vi "Configure Proxy Server.vi"(5 "proxy password":string, 7 "proxy username":string, 8 "error in":errorcluster, 9 "proxy port":u16, 10 "proxy":string, 11 "session in":refnum<class "Session.lvclass">) -> (0 "error out":errorcluster, 3 "session out":refnum<class "Session.lvclass">)   [LabVIEW 2019, in "NI_Advanced HTTP Client.lvlib" / "Session.lvclass"]
doc: "Configures the session to use a proxy server and provides the required login credentials for the proxy."
uses:
  Session.lvclass
  Session.lvclass/Session.ctl
  lvwebclient_32.dll
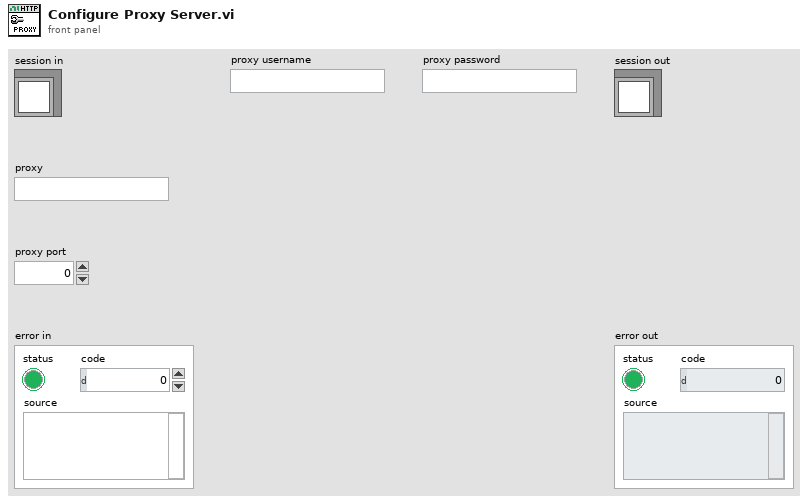
[diagram p1: front panel]
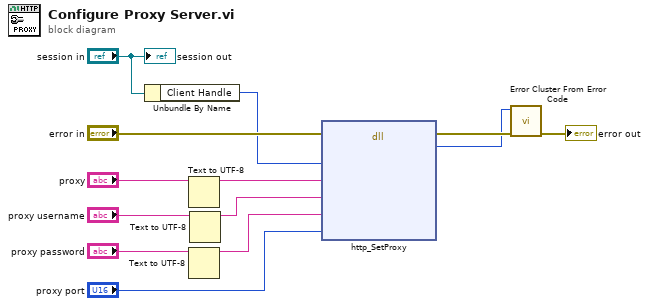
[diagram p0: block diagram]
diagram:
  n1 = Unbundle By Name("session in") -> ("Client Handle"=w8:u32)
  n2 = Text to UTF-8(11:"proxy") -> (3:w6:string)  [unwired: 2 in, 1 out]
  n3 = Text to UTF-8(11:"proxy password") -> (3:w3:string)  [unwired: 2 in, 1 out]
  n4 = Text to UTF-8(11:"proxy username") -> (3:w5:string)  [unwired: 2 in, 1 out]
  n5 = dll-call lib="C:/source/github/ni-adv-http-api/Advanced HTTP Client/lvwebclient_*.*" fn="http_SetProxy"(error in="error in", "handle"=w8, "proxy"=w6, "proxyUser"=w5, "proxyPW"=w3, "proxyPort"="proxy port") -> (error out=w9:errorcluster, "return"=w1:i32)  [unwired: 7 in, 1 out]
  n6 = call <vilib>:"Error Cluster From Error Code.vi"("error in (no error)"=w9, "error code (0)"=w1) -> ("error out"=→"error out":errorcluster)  [unwired: 7 in]
  "session out" <- "session in"
